vi "TDC_startCalibration.vi"(8 "Error In":errorcluster, 11 "Calibrate":bool) -> (0 "Error Out":errorcluster)   [LabVIEW 2011]
uses:
  tdcbase.dll
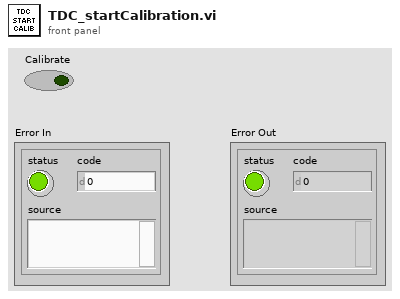
[diagram p1: front panel]
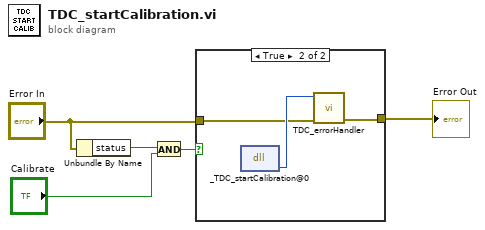
[diagram p0: block diagram]
diagram:
  n1 = Unbundle By Name("Error In") -> ("status"=w2:bool)
  n2 = And(x=w2, y="Calibrate") -> (x .and. y?=w3:bool)
  n3 = case shown="True" w3 {
    tunnel: [w6 w8] -> w5
    tunnel: "Error In" -> [w6 w7]
    frame False {
    }
    frame True {
      n4 = dll-call lib="X:/tdcbase.dll" fn="_TDC_startCalibration@0"() -> ("return type"=w9:i32)  [unwired: 3 in, 2 out]
      n5 = call "TDC_errorHandler.vi"("Error In"=w7, "TDC Return Code"=w9) -> ("Error Out"=w8:errorcluster)  [unwired: 9 in]
    }
  }
  "Error Out" <- w5
